vi "zmq version.vi"(8 "error in (no error)":errorcluster) -> (0 "error out":errorcluster, 1 "patch_ out":i32, 2 "minor_ out":i32, 3 "major_ out":i32)   [LabVIEW 2025, in "LibZMQ.lvlib"]
doc: "ZMQ_EXPORT void zmq_version (int *major_, int *minor_, int *patch_);"
uses:
  LibZMQ.lvlib
panel:
  in  "path in":path
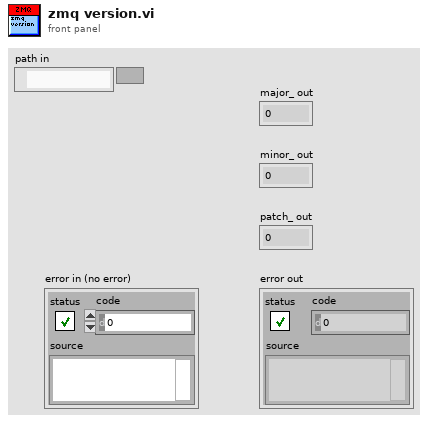
[diagram p1: front panel]
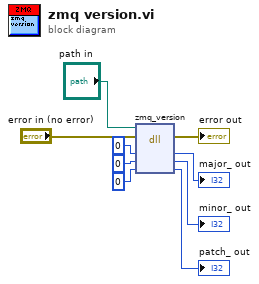
[diagram p0: block diagram]
diagram:
  n1 = dll-call lib="home/james/Documents/ZeroMQ_LV/libzmq-v143-mt-4_3_6/libzmq.so" fn="zmq_version"(path in="path in", error in="error in (no error)", "major_"=0, "minor_"=0, "patch_"=0) -> (error out=→"error out":errorcluster, "major_"=→"major_ out":i32, "minor_"=→"minor_ out":i32, "patch_"=→"patch_ out":i32)  [unwired: 2 in, 1 out]
